vi "serial pause.vi"(2 "delay (ms)":u16, 3 "Serial Port in":refnum<visa-resource-name>) -> (1 "Serial Port out":refnum<visa-resource-name>)   [LabVIEW 2012]
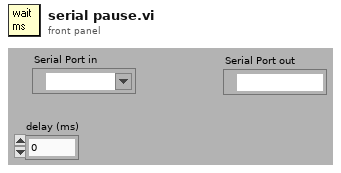
[diagram p1: front panel]
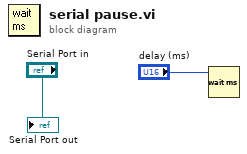
[diagram p0: block diagram]
diagram:
  n1 = Wait (ms)(milliseconds to wait="delay (ms)") -> ()  [unwired: 1 out]
  "Serial Port out" <- "Serial Port in"
